vi "File.Recursive Search.vi"(9 "Search Pattern":string, 10 "Folders":path[](array[path]), 11 "Files In":path[](array[path])) -> (2 "SubFolders":path[](array[path]), 3 "Files Out":path[](array[path]))   [LabVIEW 2018]
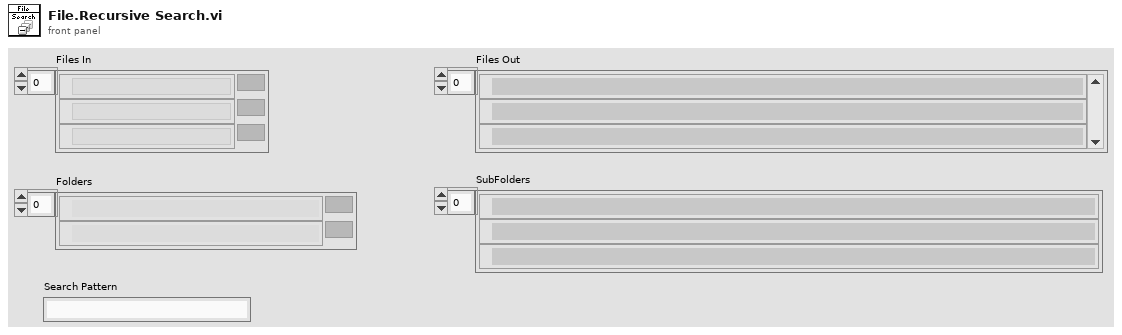
[diagram p1: front panel]
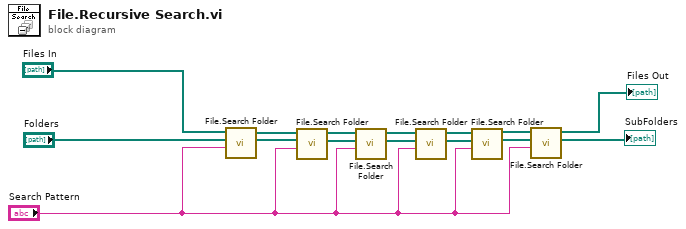
[diagram p0: block diagram]
diagram:
  n1 = call "File.Search Folder.vi"("Search Pattern"="Search Pattern", "Folders"="Folders", "Files In"="Files In") -> ("SubFolders"=w12:path[], "Files Out"=w13:path[])  [unwired: 7 in]
  n2 = call "File.Search Folder.vi"("Search Pattern"="Search Pattern", "Folders"=w12, "Files In"=w13) -> ("SubFolders"=w10:path[], "Files Out"=w11:path[])  [unwired: 7 in]
  n3 = call "File.Search Folder.vi"("Search Pattern"="Search Pattern", "Folders"=w10, "Files In"=w11) -> ("SubFolders"=w8:path[], "Files Out"=w9:path[])  [unwired: 7 in]
  n4 = call "File.Search Folder.vi"("Search Pattern"="Search Pattern", "Folders"=w8, "Files In"=w9) -> ("SubFolders"=w6:path[], "Files Out"=w7:path[])  [unwired: 7 in]
  n5 = call "File.Search Folder.vi"("Search Pattern"="Search Pattern", "Folders"=w6, "Files In"=w7) -> ("SubFolders"=w4:path[], "Files Out"=w5:path[])  [unwired: 7 in]
  n6 = call "File.Search Folder.vi"("Search Pattern"="Search Pattern", "Folders"=w4, "Files In"=w5) -> ("SubFolders"=→"SubFolders":path[], "Files Out"=→"Files Out":path[])  [unwired: 7 in]
